vi "Modify ini or conf file.vi"(8 "error in (no error)":errorcluster, 10 "VS RT EXE Path":string, 11 "Local Path to ini or conf file":path) -> (0 "error out":errorcluster, 2 "VS Already Set as Startup?":bool, 3 "Dup Path to ini or conf file":path)   [LabVIEW 2014]
doc: "Adds and removes the necessary configuration tokens to the specified file"
uses:
  <vilib>/Utility/config.llb/Read Key (String).vi
  <vilib>/Utility/config.llb/Write Key (String).vi
  <vilib>/Utility/error.llb/Error Cluster From Error Code.vi
  <vilib>/ErrorRing/Error Ring.xnode
  <vilib>/Utility/config.llb/NI_LVConfig.lvlib
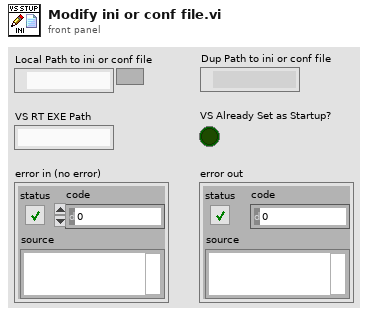
[diagram p1: front panel]
types:
  T1 = typedef "NI_LVConfig.lvlib/Config Data RefNum.ctl" = refnum<k1>
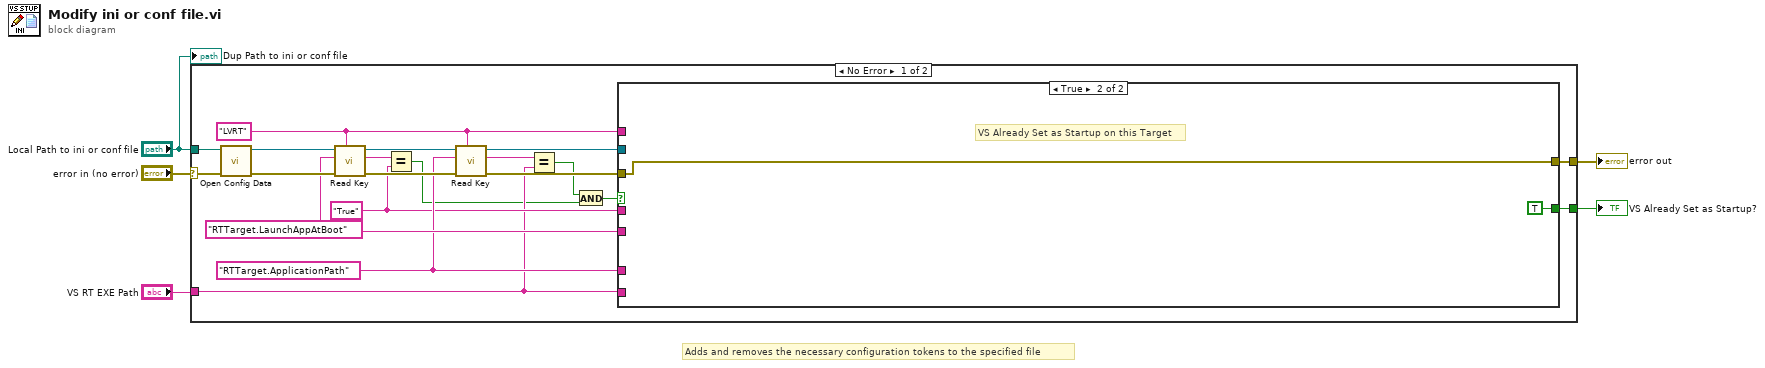
[diagram p0: block diagram]
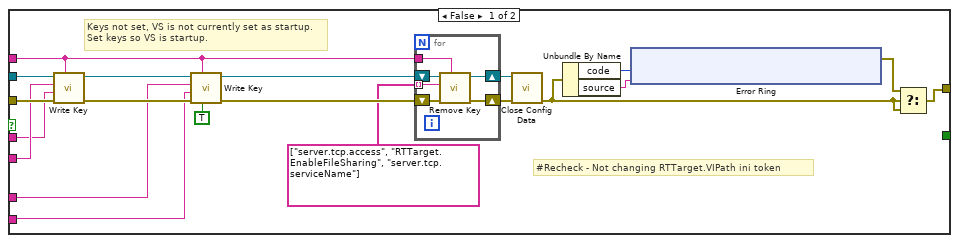
[diagram p2: hidden frame]
diagram:
  # "Adds and removes the necessary configuration tokens to the specified file"
  n1 = case shown="No Error" "error in (no error)" {
    selector: "error in (no error)" -> [w24 w62]
    tunnel: [w22 w62] -> w3
    tunnel: "Local Path to ini or conf file" -> [w25 _]
    tunnel: "VS RT EXE Path" -> [w10 _]
    tunnel: [w6 _] -> w1
    frame No Error {
      w14 = "RTTarget.ApplicationPath" ("key")
      w12 = "True" ("key")
      w16 = "RTTarget.LaunchAppAtBoot" ("key")
      w15 = "LVRT" ("section")
      n2 = call <vilib>:"Open Config Data.vi"("error in (no error)"=w24, "configuration file path"=w25) -> ("error out"=w23:errorcluster, "refnum"=w20:T1)  [unwired: 7 in, 1 out]
      n3 = call-poly <vilib>:"Read Key.vi"("section"=w15, "error in (no error)"=w23, "key"=w16, "refnum"=w20) -> ("error out"=w21:errorcluster, "value"=w13:string, "refnum out"=w18:T1)  [unwired: 4 in, 1 out]
      n4 = Equal?(x=w13, y=w12) -> (x = y?=w7:bool)
      n5 = call-poly <vilib>:"Read Key.vi"("section"=w15, "error in (no error)"=w21, "key"=w14, "refnum"=w18) -> ("error out"=w19:errorcluster, "value"=w11:string, "refnum out"=w17:T1)  [unwired: 4 in, 1 out]
      n6 = Equal?(x=w11, y=w10) -> (x = y?=w8:bool)
      n7 = And(x=w8, y=w7) -> (x .and. y?=w9:bool)
      n8 = case shown="True" w9 {
        tunnel: [w36 w61] -> w22
        tunnel: w19 -> [w32 w61]
        tunnel: w17 -> [w31 _]
        tunnel: w16 -> [w30 _]
        tunnel: w15 -> [w29 _]
        tunnel: w14 -> [w28 _]
        tunnel: w12 -> [w27 _]
        tunnel: w10 -> [w26 _]
        tunnel: [_ TRUE] -> w6
        frame False {
          # "Keys not set, VS is not currently set as startup.\nSet keys so VS is startup."
          # "#Recheck - Not changing RTTarget.VIPath ini token"
          n9 = call-poly <vilib>:"Write Key.vi"("section"=w29, "error in (no error)"=w32, "value"=w27, "key"=w30, "refnum"=w31) -> ("error out"=w44:errorcluster, "refnum out"=w45:T1)  [unwired: 4 in, 1 out]
          n10 = call-poly <vilib>:"Write Key.vi"("write raw string? (F)"=TRUE, "section"=w29, "error in (no error)"=w44, "value"=w26, "key"=w28, "refnum"=w45) -> ("error out"=w42:errorcluster, "refnum out"=w43:T1)  [unwired: 3 in, 1 out]
          n11 = for {
            tunnel: w29 -> [w57]
            shift-right: [w56] -> w41
            shift-left: w43 -> [w59]
            shift-right: [w55] -> w40
            shift-left: w42 -> [w58]
            tunnel: string[] ["server.tcp.access", "RTTarget.EnableFileSharing", "server.tcp.serviceName"] -> [w54] mode=indexing
            n12 = call <vilib>:"Remove Key.vi"("section"=w57, "error in (no error)"=w58, "key"=w54, "refnum"=w59) -> ("error out"=w55:errorcluster, "refnum out"=w56:T1)  [unwired: 5 in, 1 out]
          }
          n13 = call <vilib>:"Close Config Data.vi"("error in (no error)"=w40, "refnum"=w41) -> ("error out"=w37:errorcluster)  [unwired: 8 in, 1 out]
          n14 = Unbundle By Name(w37) -> ("code"=w35:i32, "source"=w34:string)
          n15 = xnode "Error Ring"("parameter 0"=w35, "parameter 1"=w34) -> ("error out"=w38:errorcluster)
          n16 = Select(t=w38, s=w37, f=w37) -> (s? t:f=w36:errorcluster)
        }
        frame True {
          # "VS Already Set as Startup on this Target"
        }
      }
    }
    frame Error {
    }
  }
  "error out" <- w3
  "VS Already Set as Startup?" <- w1
  "Dup Path to ini or conf file" <- "Local Path to ini or conf file"
